vi "Create File.vi"(8 "error in (no error)":errorcluster, 10 "File Name Prefix":string) -> (0 "error out":errorcluster, 3 "refnum out":refnum<file>)   [LabVIEW 2015]
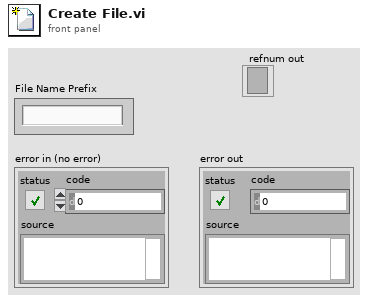
[diagram p1: front panel]
types:
  T1 = enum16{"open", "replace", "create", "open or create", "replace or create", "replace or create with confirmation"}
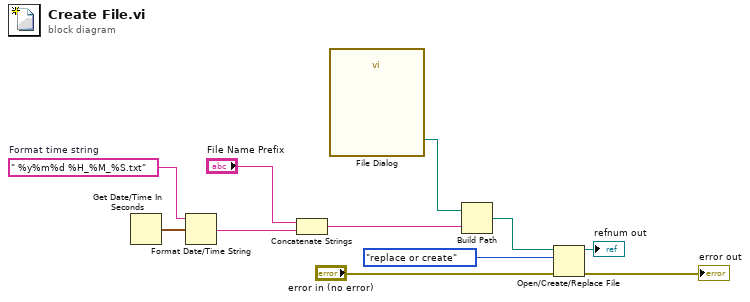
[diagram p0: block diagram]
diagram:
  w4 = " %y%m%d %H_%M_%S.txt"  # Format time string
  n1 = Get Date/Time In Seconds() -> (seconds since 1Jan1904=w2:timestamp)
  n2 = Format Date/Time String(time format string (%c)=w4, seconds (now)=w2) -> (date/time string=w5:string)  [unwired: 1 in]
  n3 = Concatenate Strings("File Name Prefix", w5) -> (w6:string)
  n4 = call "File Dialog"() -> ("selected path"=w7:path)  [unwired: 12 in, 3 out]
  n5 = Build Path(base path=w7, name or relative path=w6) -> (appended path=w8:path)
  n6 = Open/Create/Replace File(file path (use dialog)=w8, error in="error in (no error)", operation (0:open)=T1."replace or create") -> (refnum out=→"refnum out":refnum<file>, error out=→"error out":errorcluster)  [unwired: 3 in, 1 out]
